vi "Get Size of Data from TD - 1D Array (String) - Returns Correct Size.vi"() -> ()   [LabVIEW 2017, in "Composition.Tests.lvlib"]
uses:
  Composition.Tests.lvlib
  <vilib>/addons/_JKI Toolkits/Caraya/classes/Assert/Assert Equal Value_Variant.vi
  Composition/Composition.lvlib
  <vilib>/addons/_JKI Toolkits/Caraya/classes/Assert/Assert.lvclass
  <vilib>/addons/_JKI Toolkits/Caraya/classes/Test/Test.lvclass
panel:
  out "error out":errorcluster
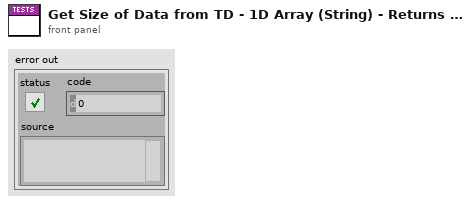
[diagram p1: front panel]
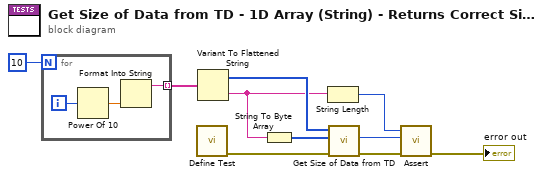
[diagram p0: block diagram]
diagram:
  n1 = for {
    N: 10 ("dimension size") -> [_]
    tunnel: [w11] -> w1 mode=indexing
    i -> [w13]
    n2 = Power Of 10(x=w13) -> (10^x=w12:dbl)
    n3 = Format Into String(w12) -> (resulting string=w11:string)  [unwired: 3 in, 1 out]
  }
  n4 = call <vilib>:"Define Test.vi"() -> ("error out"=w3:errorcluster)  [unwired: 11 in]
  n5 = Variant To Flattened String(Variant=w1) -> (data string=w7:string, 1:w10:i16[])
  n6 = String To Byte Array(string=w7) -> (unsigned byte array=w9:u8[])
  n7 = String Length(string=w7) -> (length=w4:i32)
  n8 = call "Get Size of Data from TD.vi"("error in (no error)"=w3, "Data String"=w9, "Type Descriptor"=w10) -> ("error out"=w8:errorcluster, "Size of Data"=w5:i32)  [unwired: 7 in]
  n9 = call-poly <vilib>:"Assert.vi"("error in (no error)"=w8, "Y"=w5, "X"=w4) -> ("error out"=→"error out":errorcluster)  [unwired: 8 in]
